vi "Get MLJ Stage Velocity Acceleration.vi"(8 "error in (no error)":errorcluster, 10 "Cluster in":T1, 11 ".NET Refnum in":refnum<k24>) -> (0 "error out":errorcluster, 1 "Max Vel/Accel":cluster{"maxVelocity":dbl, "acceleration":dbl}, 2 "Cluster out":T1, 3 ".NET Refnum in":refnum<k24>)   [LabVIEW 2018]
uses:
  Controls/Translation Stage Cluster.ctl
  General/Controls/Translation Stage Types.ctl
  C:/Project/SerialSectOCT - FFT GPU/SerialSectOCT/Labview Software/Thorlabs.MotionControl.Controls.dll
  Thorlabs.MotionControl.Controls.dll
  C:/Project/SerialSectOCT - FFT GPU/SerialSectOCT/Labview Software/Thorlabs.MotionControl.IntegratedStepperMotorsCLI.dll
  Thorlabs.MotionControl.IntegratedStepperMotorsCLI.dll
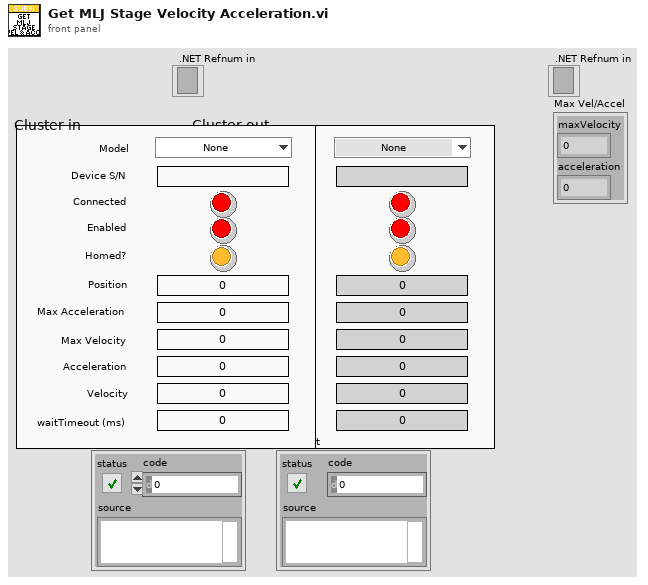
[diagram p1: front panel]
types:
  T1 = typedef "Translation Stage Cluster.ctl" = cluster{"Position":dbl, "Is.Enabled?":bool, "Is.Connected?":bool, "Device SN":string, "AccelerationMaximum":dbl, "VelocityMaximum":dbl, "Acceleration":dbl, "Velocity":dbl, "waitTimeout (ms)":i32, "Model":T2, "Is.Homed?":bool}
  T2 = typedef "Translation Stage Types.ctl" = enum16{"None", "Thorlabs LTS", "Thorlabs MLJ"}
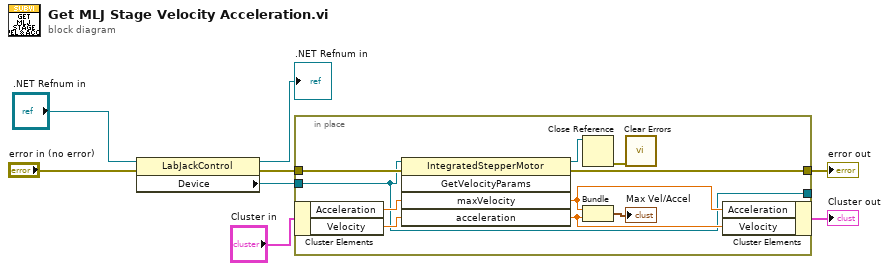
[diagram p0: block diagram]
diagram:
  n1 = property class="LabJackControl"(reference=".NET Refnum in", error in="error in (no error)") -> (reference out=→".NET Refnum in":refnum<k24>, error out=w3:errorcluster, "Device"=w1:refnum<k24>)
  n2 = in-place {
    in-place-border: [w9] -> _
    in-place-border: w3 -> [w16]
    in-place-border: [w15] -> w6
    in-place-border: w1 -> [w9]
    n3 = in-place-cluster #1("Cluster in") -> ("Acceleration"=w18:dbl, "Velocity"=w17:dbl)
    n4 = invoke class="IntegratedStepperMotor" method="GetVelocityParams"(reference=w9, error in=w16, "maxVelocity"=w18, "acceleration"=w17) -> (reference out=w13:refnum<k24>, error out=w15:errorcluster, "maxVelocity"=w12:dbl, "acceleration"=w11:dbl)  [unwired: 1 in, 1 out]
    n5 = Close Reference(reference=w13) -> (error out=w14:errorcluster)  [unwired: 1 in]
    n6 = Bundle("maxVelocity"=w12, "acceleration"=w11) -> (→"Max Vel/Accel":cluster{"maxVelocity":dbl, "acceleration":dbl})  [unwired: 1 in]
    n7 = call <vilib>:"Clear Errors.vi"("error in (no error)"=w14) -> ()  [unwired: 5 in, 2 out]
    n8 = in-place-cluster #1("Acceleration"=w12, "Velocity"=w11) -> (→"Cluster out":T1)
  }
  "error out" <- w6
